vi "Example - BMP085 (RT).vi"() -> ()   [LabVIEW 2013, in "BMP085 (RT).lvlib"]
uses:
  BMP085 (RT).lvlib
  <vilib>/myRIO/Instrument Drivers/Onboard IO/I2C/typedefs/I2C User Configuration.ctl
  <vilib>/myRIO/Instrument Drivers/Onboard IO/I2C/typedefs/I2C Transfer Rate.ctl
  <vilib>/myRIO/Instrument Drivers/Onboard IO/I2C/I2C.lvlib
panel:
  out "Pressure [hPa]":dbl(knob) scale=900.0..1100.0
  out "Temperature [°C]":dbl(slide) scale=0.0..80.0
  in  "Stop Button":bool
  # "Example: BMP085 (GY-65) - Atmospheric Pressure and Temperature Sensor"
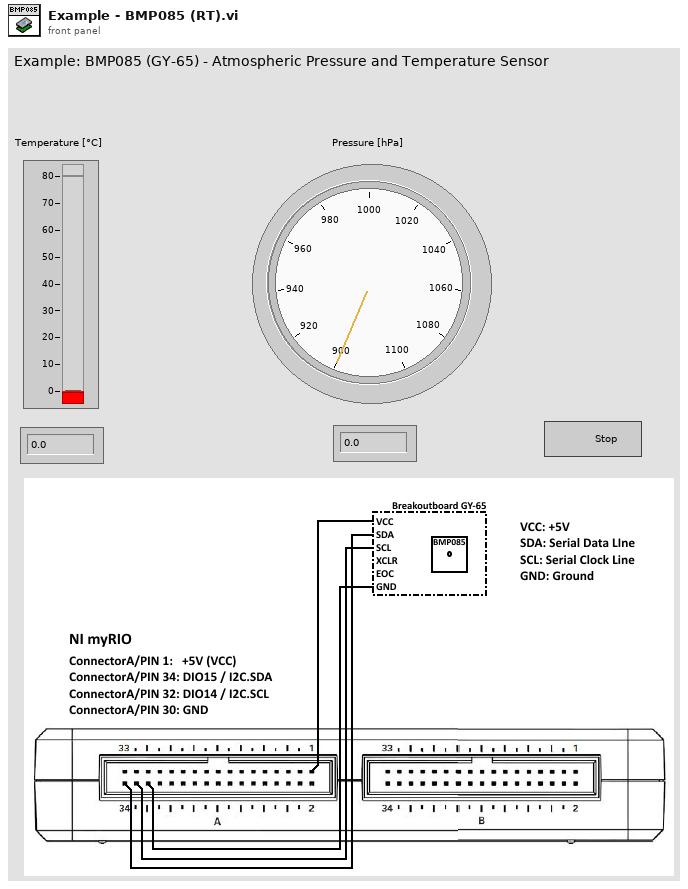
[diagram p1: front panel]
types:
  T1 = typedef "I2C.lvlib/I2C User Configuration.ctl" = cluster{"I2C Transfer Rate":T2}
  T2 = typedef "I2C.lvlib/I2C Transfer Rate.ctl" = enum16{"Standard Mode (100 kbps)", "Fast Mode (400 kbps)"}
  T3 = enum8{"ultra low power", "standard", "high resolution", "ultra high resolution"}
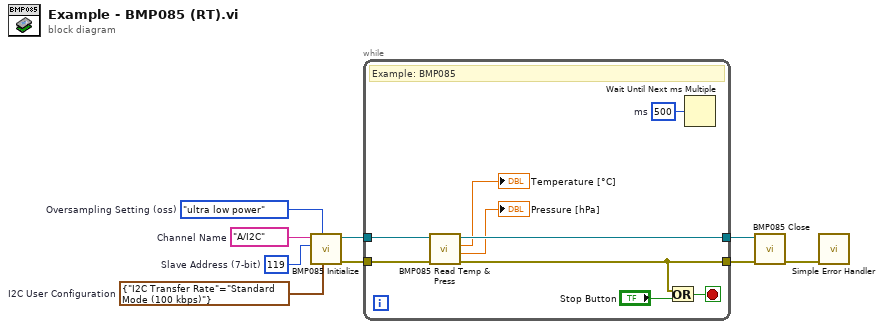
[diagram p0: block diagram]
diagram:
  w1 = T1 {"I2C Transfer Rate"=enum."Standard Mode (100 kbps)"}  # I2C User Configuration
  w4 = u8 119  # Slave Address (7-bit)
  w5 = T3."ultra low power"  # Oversampling Setting (oss)
  w6 = tag "A/I2C"  # Channel Name
  n1 = call "BMP085 Initialize.vi"("I2C User Configuration"=w1, "Oversampling Setting (oss)"=w5, "Slave Address (7-bit)"=w4, "Channel Name"=w6) -> ("error out"=w8:errorcluster, "BMP085 (GY-65) out"=w9:refnum<class "BMP085 (GY-65).lvclass">)  [unwired: 6 in]
  n2 = while {
    tunnel: w9 -> [w18]
    tunnel: [w17] -> w2
    tunnel: w8 -> [w16]
    tunnel: [w14] -> w7
    stop <- w15 stop-if-true
    w12 = u32 500  # ms
    # "Example: BMP085"
    n3 = call "BMP085 Read Temp & Press.vi"("error in (no error)"=w16, "BMP085 (GY-65) in"=w18) -> ("error out"=w14:errorcluster, "hPa"=→"Pressure [hPa]":dbl, "Temp [°C]"=→"Temperature [°C]":dbl, "BMP085 (GY-65) out"=w17:refnum<class "BMP085 (GY-65).lvclass">)  [unwired: 6 in]
    n4 = Or(x=w14, y="Stop Button") -> (x .or. y?=w15:bool)
    n5 = Wait Until Next ms Multiple(millisecond multiple=w12) -> ()  [unwired: 1 out]
  }
  n6 = call "BMP085 Close.vi"("error in (no error)"=w7, "BMP085 (GY-65) in"=w2) -> ("error out"=w3:errorcluster)  [unwired: 9 in]
  n7 = call <vilib>:"Simple Error Handler.vi"("error in (no error)"=w3) -> ()  [unwired: 4 in, 5 out]
